vi "DegreesToWindDirection.vi"(11 "Degrees":i32) -> (3 "WindDirection":string)   [LabVIEW 2015]
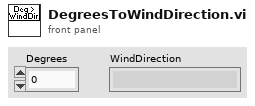
[diagram p1: front panel]
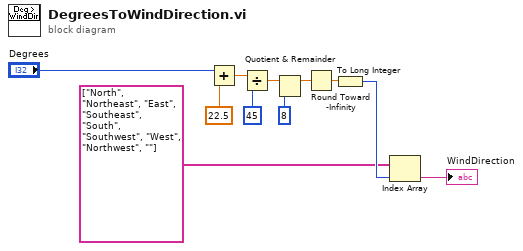
[diagram p0: block diagram]
diagram:
  n1 = Add(x="Degrees", y=22.5 ("floor(x/y)")) -> (x+y=w7:dbl)
  n2 = Divide(x=w7, y=i16 45) -> (x/y=w9:dbl)
  n3 = Quotient & Remainder(x=w9, y=i16 8) -> (x-y*floor(x/y)=w8:dbl)  [unwired: 1 out]
  n4 = Round Toward -Infinity(1:w8) -> (0:w10:dbl)
  n5 = To Long Integer(number=w10) -> (32bit integer=w11:i32)
  n6 = Index Array(array=string[] ["North", "Northeast", "East", "Southeast", "South", "Southwest", "West", "Northwest", ""], index=w11) -> (element=→"WindDirection":string)
